vi "Greater Than or Equal.vi"(9 "Semver 2":refnum<class "Semver.lvclass">, 10 "Semver 1":refnum<class "Semver.lvclass">) -> (2 "Version 1 >= Version 2":bool)   [LabVIEW 2017, in "Semver.lvlib" / "Semver.lvclass"]
uses:
  Semver.lvclass
  Semver.lvclass/Semver.ctl
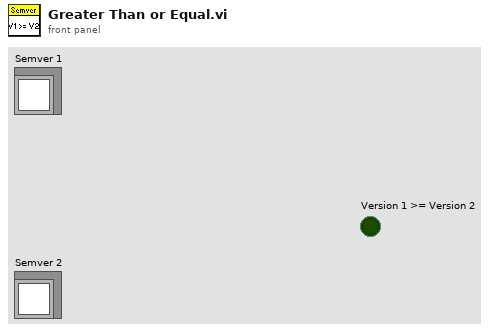
[diagram p1: front panel]
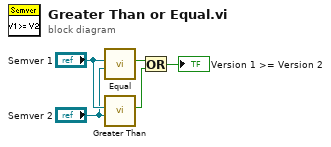
[diagram p0: block diagram]
diagram:
  n1 = call "Equal.vi"("Semver 2"="Semver 2", "Semver 1"="Semver 1") -> ("Version 1 = Version 2"=w1:bool)  [unwired: 9 in]
  n2 = call "Greater Than.vi"("Semver 2"="Semver 2", "Semver 1"="Semver 1") -> ("Version 1 > Version 2"=w5:bool)  [unwired: 9 in]
  n3 = Or(x=w1, y=w5) -> (x .or. y?=→"Version 1 >= Version 2":bool)
